vi "Main_04B.vi"() -> ()   [LabVIEW 2024]
uses:
  TypeDefs/Cluster Row-Column.ctl
panel:
  out "Answer 1998":u32
  in  "Puzzle":string="XXASMSMSXMXSMMXMAXMMMAMSAMASMSAMXMAXSXMASMAMMXXMASASXAMAMXSXMMSXSAMXSSXXMXAAXMAXMXXSXMXMMAAMMMMMMMMMMXXMSMSSSMXAAMAMMMSAMXXXXSMSAXMMXXMASMSS\nASMMAAAMAMASAXSSMMSASAMXAAAAXXXMAXXAMSASXMASMSSMSAMSAMMSXMAXSMAAMMSAMAAMSMSMSSSSXSXSMSAAXMXMAAAAMMSAMXSXMAAAAAXMAMAMAMAMMXMSASAXMXSAMXSAMXAS\nXSAMSMMSAMASXMXAAXSASXXSSMXXXMMSMSMSMAMMASASXAAXXAMXAXAMAXMASMMSMAMMSMSMAAAAAAAAASASASXSMSASXSSXSAXAMAMAMMMSMMMMAXASMSMXSAAMAMXMMAMAXXAMXMMS\nAMAMXAASMMXSAMSMMMMMMMMMAMMSMMAAAAAAXAXSAMASMSSMSAMSAMMSMMMXXAAAMXMAAAAMXMMMMSMMMMAMAMAMAMMSXMAXMASXMSSMSAMXAAASMSMXAAXAMMSMAAMAMXSMMSASXSXM\nXSAMMMMXAXSMXXAMAAXSAAXSAMASAAMMSMSM..."
  in  "Example":string="MMMSXXMASM\nMSAMXMSMSA\nAMXSXMAAMM\nMSAMASMSMX\nXMASAMXAMM\nXXAMMXXAMA\nSMSMSASXSS\nSAXAMASAAA\nMAMMMXMMMM\nMXMXAXMASX"
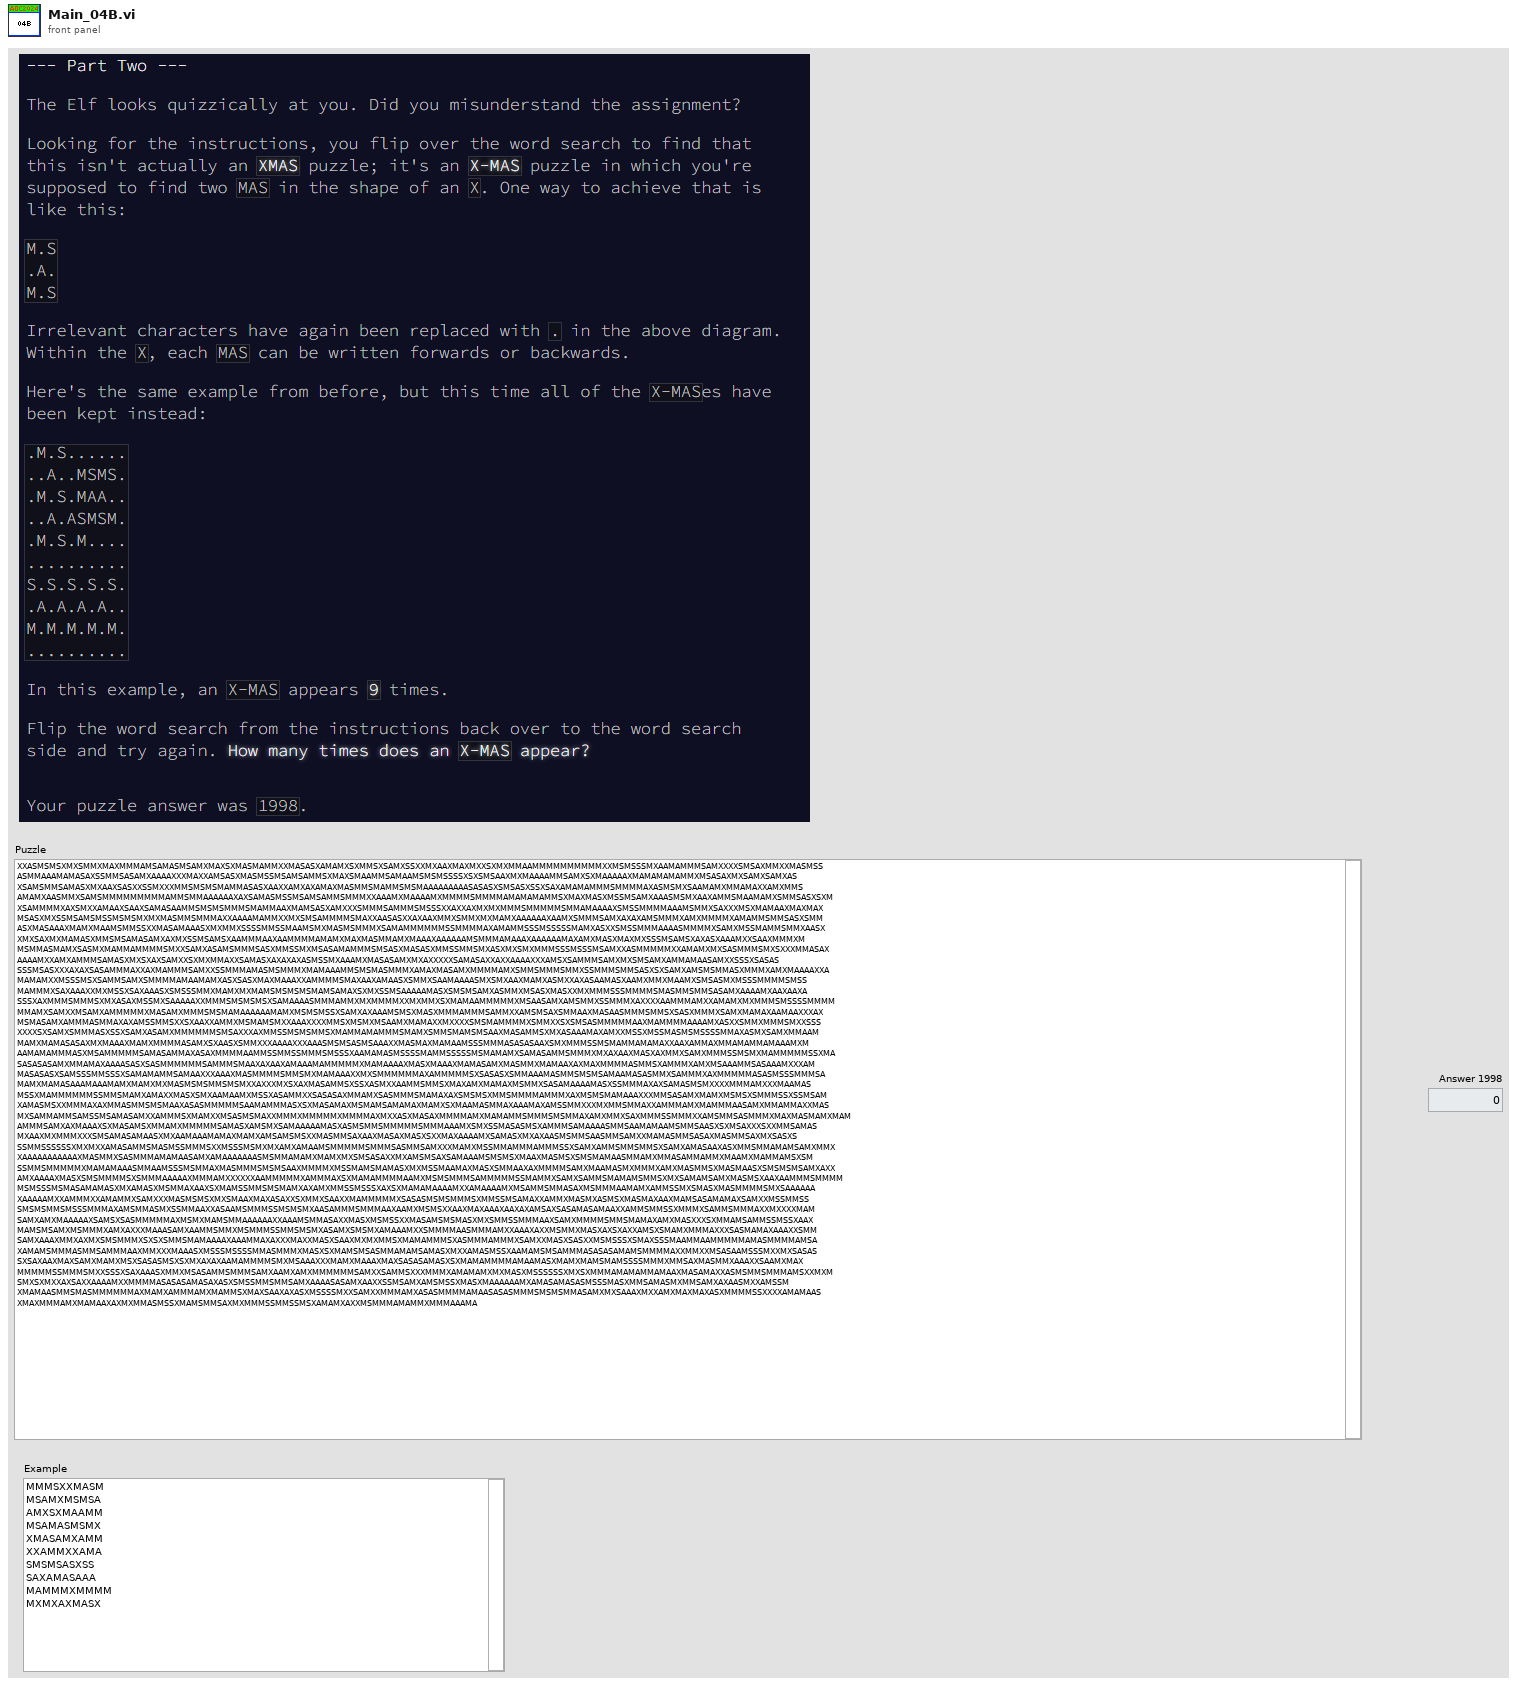
[diagram p1: front panel]
types:
  T1 = typedef "Cluster Row-Column.ctl" = cluster{"R":i32, "C":i32}
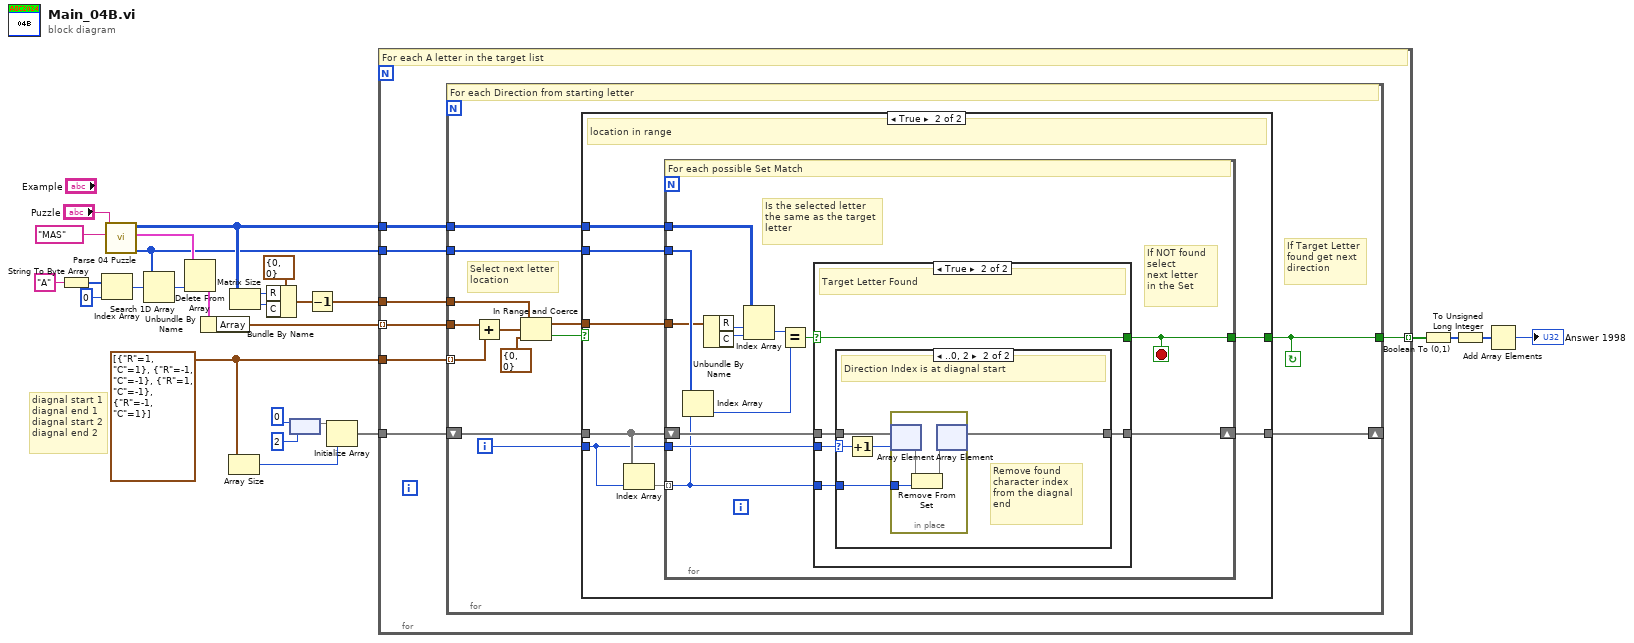
[diagram p0: block diagram]
diagram:
  w12 = T1[] [{"R"=1, "C"=1}, {"R"=-1, "C"=-1}, {"R"=1, "C"=-1}, {"R"=-1, "C"=1}]
  # "diagnal start 1\ndiagnal end 1\ndiagnal start 2\ndiagnal end 2"
  n1 = String To Byte Array(string="A") -> (unsigned byte array=w15:u8[])
  n2 = Index Array(array=w15, index=0) -> (element=w6:u8)
  n3 = call "Parse 04 Puzzle.vi"("Target Letters"="MAS", "Puzzle"="Puzzle") -> ("Axcii Target Letters Out"=w1:u8[], "Letter Location Array Out"=w2:cluster{"Array":T1[]}[], "Ascii Byte Array Out"=w3:u8[][])  [unwired: 7 in]
  n4 = Search 1D Array(1D array=w1, element=w6) -> (index of element=w13:i32)  [unwired: 1 in]
  n5 = Delete From Array(array=w2, index=w13) -> (deleted portion=w27:cluster{"Array":T1[]})  [unwired: 1 in, 1 out]
  n6 = Unbundle By Name(w27) -> ("Array"=w26:T1[])
  n7 = Array Size(array=w12) -> (size(s)=w11:i32)
  n8 = Matrix Size(0:w3) -> (1:w24:i32, 2:w23:i32)
  n9 = Bundle By Name(cluster=T1 {"R"=0, "C"=0}, "R"=w24, "C"=w23) -> (w22:T1)
  n10 = node(0 ("index"), 2 ("index")) -> (w7:set{i32})
  n11 = Decrement(x=w22) -> (x-1=w21:T1)
  n12 = Initialize Array(w7, w11) -> (w10:set{i32}[])
  n13 = for {
    tunnel: w26 -> [w30] mode=indexing
    tunnel: w3 -> [w34]
    tunnel: w12 -> [w32]
    tunnel: w21 -> [w31]
    tunnel: w1 -> [w33]
    tunnel: [w29] -> w19 mode=indexing
    tunnel: w10 -> [w28]
    # "For each A letter in the target list"
    n14 = for {
      tunnel: w34 -> [w47]
      tunnel: w31 -> [w43]
      tunnel: w33 -> [w46]
      tunnel: w32 -> [w44] mode=indexing
      tunnel: [w37] -> w29
      tunnel: w30 -> [w45]
      shift-right: [w36] -> _
      shift-left: w28 -> [w38]
      i -> [w35]
      stop <- w37 continue-if-true
      # "If Target Letter\nfound get next\ndirection"
      # "Select next letter\nlocation"
      # "For each Direction from starting letter"
      n15 = Add(x=w45, y=w44) -> (x+y=w42:T1)
      n16 = In Range and Coerce(upper limit=w43, x=w42, lower limit=T1 {"R"=0, "C"=0}) -> (coerced(x)=w40:T1, In Range?=w39:bool)
      n17 = case shown="True" w39 {
        selector: w39 -> [w49 _]
        tunnel: w47 -> [_ w57]
        tunnel: w46 -> [_ w56]
        tunnel: w40 -> [_ w54]
        tunnel: [w49 w55] -> w37
        tunnel: w38 -> [w48 w52]
        tunnel: w35 -> [_ w50]
        tunnel: [w48 w51] -> w36
        frame False {
          # "location NOT in range"
        }
        frame True {
          # "location in range"
          n18 = Index Array(array=w52, index=w50) -> (element=w53:set{i32})
          n19 = for {
            tunnel: w57 -> [w70]
            tunnel: w56 -> [w69]
            tunnel: [w61] -> w55
            tunnel: w54 -> [w64]
            tunnel: w53 -> [w59] mode=indexing
            shift-right: [w58] -> w51
            shift-left: w52 -> [w62]
            tunnel: w50 -> [w60]
            stop <- w61 stop-if-true
            # "If NOT found\nselect\nnext letter\nin the Set"
            # "Is the selected letter\nthe same as the target\nletter"
            # "For each possible Set Match"
            n20 = Index Array(array=w69, index=w59) -> (element=w65:u8)
            n21 = Unbundle By Name(w64) -> ("R"=w68:i32, "C"=w67:i32)
            n22 = Index Array(array=w70, index (row)=w68, index (col)=w67) -> (element=w66:u8)
            n23 = Equal?(x=w66, y=w65) -> (x = y?=w63:bool)
            n24 = case shown="True" w63 {
              selector: w63 -> [w72 w73]
              tunnel: w62 -> [w71 w75]
              tunnel: [w72 w73] -> w61
              tunnel: w60 -> [_ w77]
              tunnel: w59 -> [_ w76]
              tunnel: [w71 w74] -> w58
              frame False {
              }
              frame True {
                # "Target Letter Found"
                n25 = case shown="..0, 2" w77 {
                  selector: w77 -> [_ w81]
                  tunnel: w76 -> [_ w83]
                  tunnel: w75 -> [w78 w82]
                  tunnel: [w78 w80] -> w74
                  frame 1, 3.. {
                    # "Direction Index is NOT at diagnal start"
                  }
                  frame ..0, 2 {
                    # "Remove found\ncharacter index\nfrom the diagnal\nend"
                    # "Direction Index is at diagnal start"
                    n26 = Increment(x=w81) -> (x+1=w79:i32)
                    n27 = in-place {
                      in-place-border: w83 -> [w86]
                      n28 = in-place-array #1(w82, w79) -> (w85:set{i32})
                      n29 = Remove From Set(10:w86, 11:w85) -> (3:w84:set{i32})  [unwired: 1 out]
                      n30 = in-place-array #1(w84) -> (w80:set{i32}[])  [unwired: 1 out]
                    }
                  }
                }
              }
            }
          }
        }
      }
    }
  }
  n31 = Boolean To (0,1)(Boolean=w19) -> (0, 1=w18:i16[])
  n32 = To Unsigned Long Integer(number=w18) -> (unsigned 32bit integer=w17:u32[])
  n33 = Add Array Elements(numeric array=w17) -> (sum=→"Answer 1998":u32)
